vi "test.vi"() -> ()   [LabVIEW 2017]
panel:
  out "checksum error":bool
  in  "stop":bool
  out "Waveform Chart":T1(graph)
  in  "port":refnum<visa-resource-name>="ASRL2::INSTR"
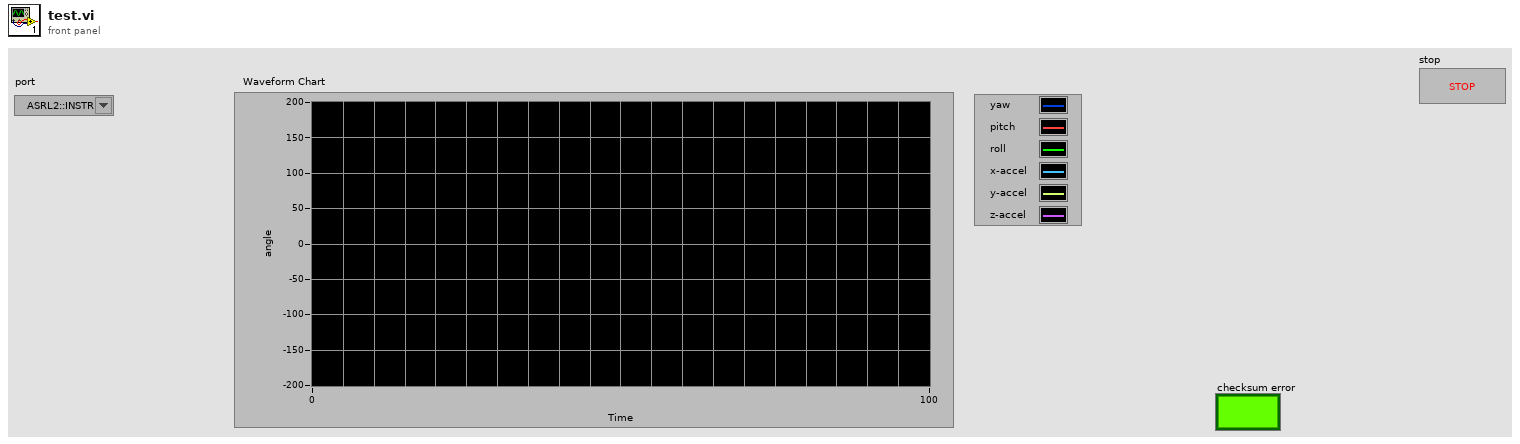
[diagram p1: front panel]
types:
  T1 = cluster{"yaw":dbl, "pitch":dbl, "roll":dbl, "x-accel":dbl, "y-accel":dbl, "z-accel":dbl}
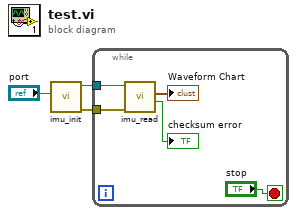
[diagram p0: block diagram]
diagram:
  n1 = call "imu_init.vi"("port"="port") -> ("error out"=w1:errorcluster, "VISA resource name out"=w3:refnum<visa-resource-name>)  [unwired: 9 in]
  n2 = while {
    tunnel: w3 -> [w8]
    tunnel: w1 -> [w7]
    stop <- "stop" stop-if-true
    n3 = call "imu_read.vi"("error in"=w7, "VISA resource name"=w8) -> ("checksum error"=→"checksum error":bool, "data"=→"Waveform Chart":T1)  [unwired: 6 in, 2 out]
  }
